vi "Build Attitude Text.vi"(10 "angle units":T1, 11 "attitude (rad)":T2) -> (3 "text":string)   [LabVIEW 2017, in "NI_Robotics_Attitude Picture.lvlib"]
uses:
  <vilib>/robotics/Controls/Attitude Indicator/Attitude Picture/NI_Robotics_Attitude Picture.lvlib
  <vilib>/robotics/Controls/Attitude Indicator/Attitude Picture/Attitude.ctl
  <vilib>/robotics/Controls/Utilities/Angle Units.ctl
  <vilib>/Utility/AngleManip/Radians to Degrees (Scalar DBL).vi
  <vilib>/Utility/AngleManip/NI_AngleManipulation.lvlib
  <vilib>/robotics/Controls/Utilities/NI_Robotics_Control Utilities.lvlib
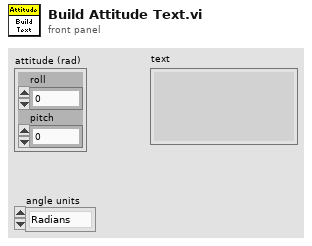
[diagram p1: front panel]
types:
  T1 = typedef "NI_Robotics_Control Utilities.lvlib/Angle Units.ctl" = enum16{"Radians", "Degrees"}
  T2 = typedef "NI_Robotics_Attitude Picture.lvlib/Attitude.ctl" = cluster{"roll":dbl, "pitch":dbl}
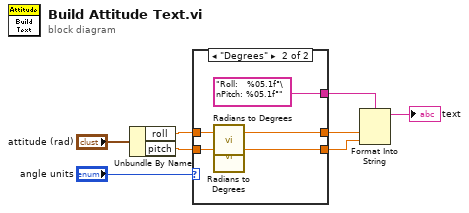
[diagram p0: block diagram]
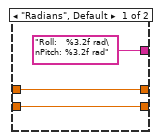
[diagram p2: hidden frame]
diagram:
  n1 = Unbundle By Name("attitude (rad)") -> ("roll"=w6:dbl, "pitch"=w5:dbl)
  n2 = case shown="\"Degrees\"" "angle units" {
    tunnel: w6 -> [w11 w16]
    tunnel: w5 -> [w10 w15]
    tunnel: [w11 w14] -> w4
    tunnel: [w10 w13] -> w3
    tunnel: ["Roll:   %3.2f rad\nPitch: %3.2f rad" "Roll:   %05.1f°\nPitch: %05.1f°"] -> w1
    frame "Radians", Default {
    }
    frame "Degrees" {
      n3 = call-poly <vilib>:"Radians to Degrees.vi"("angle (rad)"=w16) -> ("angle (deg)"=w14:dbl)  [unwired: 2 in]
      n4 = call-poly <vilib>:"Radians to Degrees.vi"("angle (rad)"=w15) -> ("angle (deg)"=w13:dbl)  [unwired: 2 in]
    }
  }
  n5 = Format Into String(format string=w1, w4, w3) -> (resulting string=→"text":string)  [unwired: 2 in, 1 out]
